vi "Read Self Attributes.vi"(7 "Actor in":refnum<class "Actor.lvclass">) -> (2 "Self Attributes":refnum<class "Attributes.lvclass">)   [LabVIEW 2020, in "jettl.lvlib"]
uses:
  jettl.lvlib
  Attributes/Attributes.lvclass
  Actor/Actor.lvclass
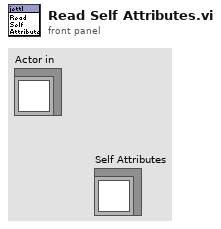
[diagram p1: front panel]
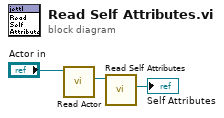
[diagram p0: block diagram]
diagram:
  n1 = call-dynamic "Read Actor.vi"("Actor in"="Actor in") -> ("Actor"=w2:refnum<class "Actor.lvclass">)  [unwired: 10 in]
  n2 = call-dynamic "Read Self Attributes.vi"("Actor in"=w2) -> ("Self Attributes"=→"Self Attributes":refnum<class "Attributes.lvclass">)  [unwired: 10 in]
